vi "Set Protocol_ex.vi"() -> ()   [LabVIEW 2019]
uses:
  Addon/Support Libraries/Protocols.lvlibp/Protocol Parent/Protocol Parent.lvclass
  <vilib>/NI VeriStand/Custom Device API/Custom Device Item Ref.ctl
  Scripting API/Scripting API.lvlib
  <vilib>/NI VeriStand/Custom Device API/Custom Device API.lvlib
panel:
  out "instrument addon refnum out":T1=18446744073709551615 format="%.0x"
  out "error out":errorcluster
  in  "instrument addon refnum in":T1=18446744073709551615 format="%.0x"
  in  "protocol":refnum<class "Protocol Parent.lvclass">
  in  "error in (no error)":errorcluster
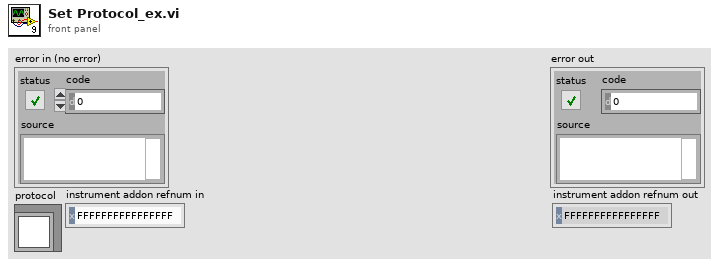
[diagram p1: front panel]
types:
  T1 = typedef "Custom Device API.lvlib/Custom Device Item Ref.ctl" = u64
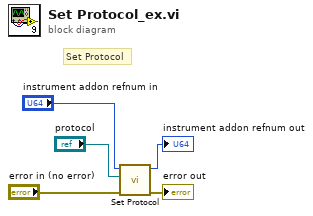
[diagram p0: block diagram]
diagram:
  # "Set Protocol"
  n1 = call "Set Protocol.vi"("error in (no error)"="error in (no error)", "protocol"="protocol", "instrument addon refnum in"="instrument addon refnum in") -> ("error out"=→"error out":errorcluster, "instrument addon refnum out"=→"instrument addon refnum out":T1)  [unwired: 7 in]
